vi "Add Dynamic Node Pages in XML.vi"(6 "XML Path":path, 7 "Add Separator?":bool, 8 "error in":errorcluster, 10 "Custom Device Name":string, 11 "Page Properties":T1) -> (0 "error out":errorcluster)   [LabVIEW 2026, in "NIVS_CDEW_MetaDataObj.lvclass"]
uses:
  NIVS_CDEW_MetaDataObj.lvclass
  Types/Page Properties.ctl
  Types/Page Types.ctl
  <vilib>/xml/Load XML File.vi
  NIVS_CDEW_MetaDataObj.lvclass/NIVS_CDEW_MetaDataObj.ctl
  <vilib>/xml/NI_XML.lvlib
  <resource>/objmgr/DOMUserDefRef.rc
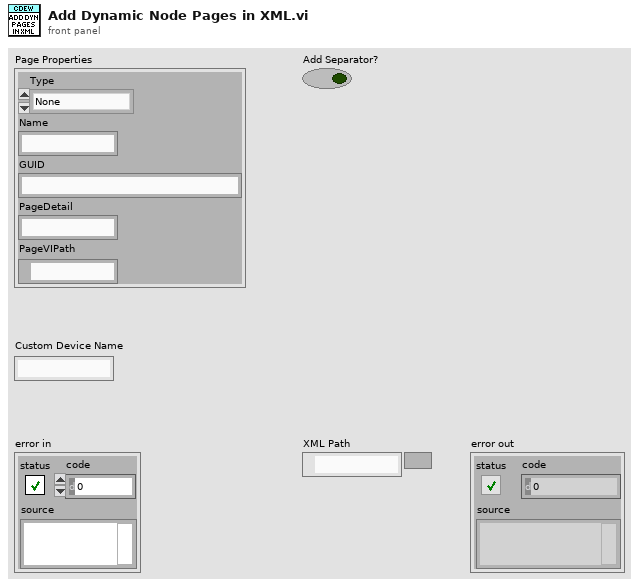
[diagram p1: front panel]
types:
  T1 = typedef "NIVS_CDEW_MetaDataObj.lvclass/Page Properties.ctl" = cluster{"Type":T2, "Name":string, "GUID":string, "PageDetail":string, "PageVIPath":path}
  T2 = typedef "NIVS_CDEW_MetaDataObj.lvclass/Page Types.ctl" = enum16{"None", "CustomDevice", "Channel", "Waveform", "Section", "DynamicChannel", "DynamicWaveform", "DynamicSection"}
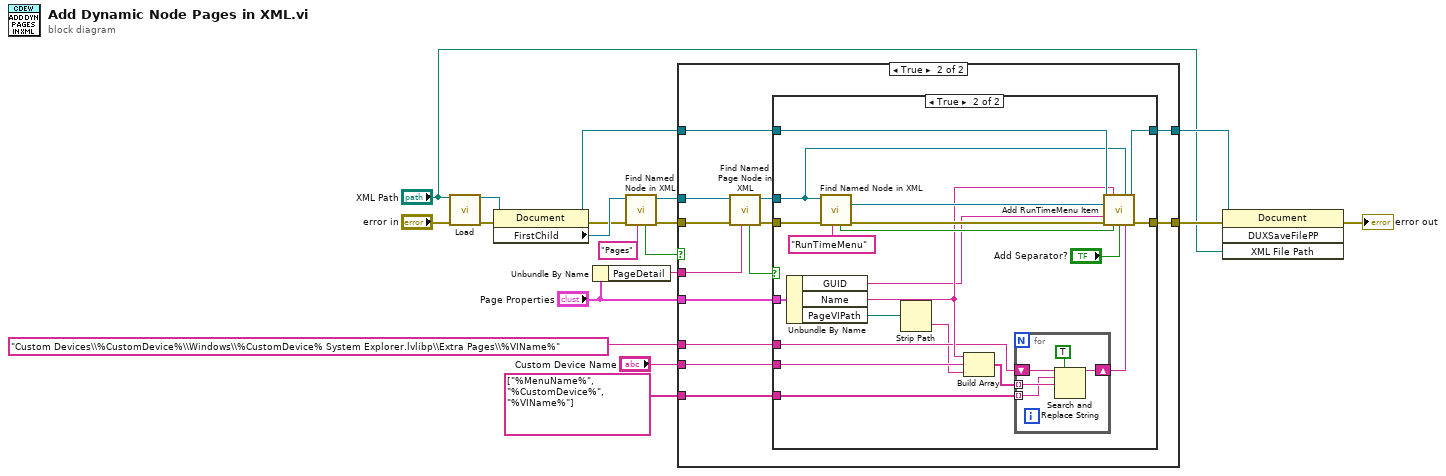
[diagram p0: block diagram]
diagram:
  n1 = call-poly <vilib>:"Load.vi"("path to XML document"="XML Path", "error in (no error)"="error in") -> ("DOM document out"=w14:refnum<k20>, "error out"=w19:errorcluster)  [unwired: 11 in, 1 out]
  n2 = property class="Document"(reference=w14, error in=w19) -> (reference out=w10:refnum<k20>, error out=w15:errorcluster, "FirstChild"=w16:refnum<k20>)
  n3 = Unbundle By Name("Page Properties") -> ("PageDetail"=w1:string)
  n4 = call "Find Named Node in XML.vi"("Node Name"="Pages", "error in"=w15, "Node in"=w16) -> ("error out"=w17:errorcluster, "Matched Node Ref"=w18:refnum<k20>, "Node Found?"=w12:bool)  [unwired: 6 in]
  n5 = case shown="True" w12 {
    tunnel: w18 -> [_ w22]
    tunnel: w17 -> [w21 w23]
    tunnel: [w21 w34] -> w9
    tunnel: w1 -> [_ w24]
    tunnel: w10 -> [w20 w33]
    tunnel: [w20 w32] -> w7
    tunnel: "Page Properties" -> [_ w31]
    tunnel: "Custom Device Name" -> [_ w30]
    tunnel: "Custom Devices\\%CustomDevice%\\Windows\\%CustomDevice% System Explorer.lvlibp\\Extra Pages\\%VIName%" -> [_ w29]
    tunnel: string[] ["%MenuName%", "%CustomDevice%", "%VIName%"] -> [_ w28]
    frame False {
    }
    frame True {
      n6 = call "Find Named Page Node in XML.vi"("Page Name"=w24, "error in"=w23, "Node in"=w22) -> ("error out"=w27:errorcluster, "Matched Node Ref"=w25:refnum<k20>, "Node Found?"=w26:bool)  [unwired: 6 in]
      n7 = case shown="True" w26 {
        tunnel: w27 -> [w36 w56]
        tunnel: [w36 w54] -> w34
        tunnel: w33 -> [w35 w50]
        tunnel: [w35 w51] -> w32
        tunnel: w31 -> [_ w49]
        tunnel: w30 -> [_ w47]
        tunnel: w29 -> [_ w44]
        tunnel: w28 -> [_ w43]
        tunnel: w25 -> [_ w38]
        frame False {
        }
        frame True {
          n8 = Unbundle By Name(w49) -> ("GUID"=w41:string, "Name"=w48:string, "PageVIPath"=w39:path)
          n9 = call "Find Named Node in XML.vi"("Node Name"="RunTimeMenu" ("y"), "error in"=w56, "Node in"=w38) -> ("error out"=w55:errorcluster, "Matched Node Ref"=w53:refnum<k20>, "Node Found?"=w52:bool)  [unwired: 6 in]
          n10 = Strip Path(path=w39) -> (name=w40:string)  [unwired: 1 out]
          n11 = Build Array(w48, w47, w40) -> (w45:string[])
          n12 = for {
            shift-right: [w60] -> w46
            shift-left: w44 -> [w61]
            tunnel: w45 -> [w58] mode=indexing
            tunnel: w43 -> [w57] mode=indexing
            n13 = Search and Replace String(replace all?=TRUE ("replace all? (F)"), input string=w61, search string=w57, replace string=w58) -> (result string=w60:string)  [unwired: 4 in, 3 out]
          }
          n14 = call "Add RunTimeMenu Item.vi"("Document In"=w50, "Name"=w48, "Node In"=w38, "New Element In"=w53, "GUID"=w41, "error in"=w55, "RunTimeMenu Found?"=w52, "Add Separator?"="Add Separator?", "Path"=w46) -> ("Document out"=w51:refnum<k20>, "error out"=w54:errorcluster)  [unwired: 5 in]
        }
      }
    }
  }
  n15 = invoke class="Document" method="DUXSaveFilePP"(reference=w7, error in=w9, "XML File Path"="XML Path") -> (error out=→"error out":errorcluster)  [unwired: 1 in, 3 out]
